vi "UHR-Fleezers Control (host) - 11.9c.vi"() -> ()   [LabVIEW 2014] (continued)
                              n670 = flat-sequence {
                                tunnel: w977 -> [w980]
                                tunnel: [w979] -> w976
                                tunnel: ["N Array El"] -> w975
                                tunnel: w976 -> [w994]
                                tunnel: w975 -> [w990]
                                frame #0 {
                                n671 = Multiply(x="Yank Delay (s)", y=1000.0) -> (x*y=w983:dbl)
                                n672 = Quotient & Remainder(x=w980, y="N Array El") -> (x-y*floor(x/y)=w979:u8)  [unwired: 1 out]
                                n673 = Wait (ms)(milliseconds to wait=w983) -> ()  [unwired: 1 out]
                                }
                                frame #1 {
                                n674 = Random Number (0-1)() -> (number: 0 to 1=w991:dbl)
                                n675 = Multiply(x=w990, y=w991) -> (x*y=w989:dbl)
                                n676 = Round Toward -Infinity(1:w989) -> (0:w988:dbl)
                                n677 = Select(t=w988, s="Random Choice", f=w994) -> (s? t:f=w992:dbl)
                                n678 = Select(t="Yank to Trap D (MHz)", s="Yank to which?", f="Yank to SP") -> (s? t:f=w985:dbl[])
                                n679 = Index Array(array=w985, index=w992) -> (element=w995:dbl)
                                n680 = case shown="False" "Yank to which?" {
                                tunnel: w995 -> [w996 w1023]
                                frame False {
                                n681 = flat-sequence {
                                tunnel: w996 -> [w997]
                                frame #0 {
                                n682 = property on="Trap Pos FB SP" class="DigNum (strict)"("Val(Sgnl)"=w997) -> ()  [unwired: 2 in, 2 out]
                                }
                                frame #1 {
                                n683 = Wait (ms)(milliseconds to wait=u32 700) -> ()  [unwired: 1 out]
                                }
                                frame #2 {
                                n684 = local read "Action (%)"() -> (w1002:dbl)
                                n685 = Absolute Value(x=w1002) -> (abs(x)=w1001:dbl)
                                n686 = Greater?(x=w1001, y=70.0) -> (0:w999:bool)
                                n687 = property on="Remove Action Offset" class="Bool (strict)"("Val(Sgnl)"=w999) -> ()  [unwired: 2 in, 2 out]
                                }
                                frame #3 {
                                n688 = for {
                                N: 4 -> [_]
                                n689 = flat-sequence {
                                frame #0 {
                                n690 = Wait (ms)(milliseconds to wait=u32 500) -> ()  [unwired: 1 out]
                                }
                                frame #1 {
                                n691 = local read "Action (%)"() -> (w1008:dbl)
                                n692 = Absolute Value(x=w1008) -> (abs(x)=w1007:dbl)
                                n693 = Greater?(x=w1007, y=70.0) -> (0:w1005:bool)
                                n694 = property on="Remove Action Offset" class="Bool (strict)"("Val(Sgnl)"=w1005) -> ()  [unwired: 2 in, 2 out]
                                }
                                }
                                }
                                }
                                frame #4 {
                                n695 = local read "Shift confocal"() -> (w1012:bool)
                                n696 = local read "Mean"() -> (w1015:dbl)
                                n697 = Greater?(x=w1015, y=11.0) -> (0:w1011:bool)
                                n698 = Not(x=w1011) -> (.not. x?=w1010:bool)
                                n699 = And(x=w1010, y=w1012) -> (x .and. y?=w1009:bool)
                                n700 = And(x=w1011, y=w1012) -> (x .and. y?=w1013:bool)
                                n701 = case shown="True" w1013 {
                                frame False {
                                }
                                frame True {
                                n702 = local read "Confocal X 2 (V)"() -> (w1018:dbl)
                                n703 = local read "Confocal Y 2 (V)"() -> (w1019:dbl)
                                n704 = property on="AO2" class="Slide (strict)"("Val(Sgnl)"=w1018) -> ()  [unwired: 2 in, 2 out]
                                n705 = property on="AO1" class="Slide (strict)"("Val(Sgnl)"=w1019) -> ()  [unwired: 2 in, 2 out]
                                }
                                }
                                n706 = case shown="True" w1009 {
                                frame False {
                                }
                                frame True {
                                n707 = local read "Confocal X 1 (V)"() -> (w1016:dbl)
                                n708 = local read "Confocal Y 1 (V)"() -> (w1017:dbl)
                                n709 = property on="AO1" class="Slide (strict)"("Val(Sgnl)"=w1017) -> ()  [unwired: 2 in, 2 out]
                                n710 = property on="AO2" class="Slide (strict)"("Val(Sgnl)"=w1016) -> ()  [unwired: 2 in, 2 out]
                                }
                                }
                                }
                                frame #5 {
                                n711 = Wait (ms)(milliseconds to wait=u32 1500) -> ()  [unwired: 1 out]
                                }
                                frame #6 {
                                n712 = property on="Remove Offset" class="Bool (strict)"("Val(Sgnl)"=TRUE ("Value (Signaling)")) -> ()  [unwired: 2 in, 2 out]
                                n713 = property on="Rem fb disp offset" class="Bool (strict)"("Val(Sgnl)"=TRUE ("Value (Signaling)")) -> ()  [unwired: 2 in, 2 out]
                                }
                                }
                                }
                                frame True {
                                n714 = flat-sequence {
                                tunnel: w1023 -> [w1024]
                                frame #0 {
                                n715 = property on="Trap D (MHz)" class="DigNum (strict)"("Val(Sgnl)"=w1024) -> ()  [unwired: 2 in, 2 out]
                                }
                                frame #1 {
                                n716 = Wait (ms)(milliseconds to wait=u32 500) -> ()  [unwired: 1 out]
                                }
                                frame #2 {
                                n717 = local read "Shift confocal"() -> (w1028:bool)
                                n718 = local read "Mean"() -> (w1026:dbl)
                                n719 = Greater?(x=w1026, y=11.0) -> (0:w1029:bool)
                                n720 = Not(x=w1029) -> (.not. x?=w1030:bool)
                                n721 = And(x=w1030, y=w1028) -> (x .and. y?=w1032:bool)
                                n722 = And(x=w1029, y=w1028) -> (x .and. y?=w1031:bool)
                                n723 = case shown="True" w1031 {
                                frame False {
                                }
                                frame True {
                                n724 = local read "Confocal Y 2 (V)"() -> (w1036:dbl)
                                n725 = local read "Confocal X 2 (V)"() -> (w1035:dbl)
                                n726 = property on="AO1" class="Slide (strict)"("Val(Sgnl)"=w1036) -> ()  [unwired: 2 in, 2 out]
                                n727 = property on="AO2" class="Slide (strict)"("Val(Sgnl)"=w1035) -> ()  [unwired: 2 in, 2 out]
                                }
                                }
                                n728 = case shown="True" w1032 {
                                frame False {
                                }
                                frame True {
                                n729 = local read "Confocal X 1 (V)"() -> (w1033:dbl)
                                n730 = local read "Confocal Y 1 (V)"() -> (w1034:dbl)
                                n731 = property on="AO2" class="Slide (strict)"("Val(Sgnl)"=w1033) -> ()  [unwired: 2 in, 2 out]
                                n732 = property on="AO1" class="Slide (strict)"("Val(Sgnl)"=w1034) -> ()  [unwired: 2 in, 2 out]
                                }
                                }
                                }
                                }
                                }
                                }
                                }
                              }
                            }
                            frame "Raster" {
                              n733 = property on="Trap Raster Scan" class="Bool (strict)"("Val(Sgnl)"=TRUE ("Value (Signaling)")) -> ()  [unwired: 2 in, 2 out]
                            }
                          }
                          n734 = local read "Time (s)"() -> (w969:dbl)
                          "Fl. High" <- TRUE ("Yanking")
                        }
                        frame #1 {
                          n735 = local read "Auto F Reset"() -> (w1038:bool)
                          n736 = case shown="True" w1038 {
                            tunnel: w1043 -> [_ w1047]
                            tunnel: w1042 -> [_ w1046]
                            tunnel: w1041 -> [_ w1045]
                            tunnel: w1039 -> [_ w1044]
                            frame False {
                            }
                            frame True {
                              n737 = node-c288() -> (w1049:T22)  [unwired: 4 out]
                              n738 = timed-loop {
                                timing: w1049 -> [_]
                                timing-out: [_] -> w1048
                                tunnel: w1047 -> [w1067]
                                tunnel: w1046 -> [w1066]
                                tunnel: w1045 -> [w1065]
                                tunnel: w1044 -> [w1064]
                                stop <- w1050 stop-if-true
                                n739 = node-c288() -> ()  [unwired: 2 out]
                                n740 = local read "Fl. D Thresh. (kHz)"() -> (w1058:dbl)
                                n741 = local read "Fl. Triggered..."() -> (w1063:bool)
                                n742 = local read "Delta Fl. 1"() -> (w1054:dbl)
                                n743 = local read "Delta Fl. 2"() -> (w1052:dbl)
                                n744 = local read "Stop All"() -> (w1061:bool)
                                n745 = local read "APD to Watch"() -> (w1053:bool)
                                n746 = Select(t=w1054, s=w1053, f=w1052) -> (s? t:f=w1051:dbl)
                                n747 = Not(x=w1063) -> (.not. x?=w1062:bool)
                                n748 = Multiply(x=w1058, y=1000.0) -> (x*y=w1057:dbl)
                                n749 = Negate(x=w1057) -> (-x=w1056:dbl)
                                n750 = Less?(x=w1051, y=w1056) -> (x < y?=w1060:bool)
                                n751 = Compound Arithmetic op=OR(w1060, w1061, w1062, "Reset Force") -> (w1050:bool)
                                n752 = case shown="True" w1050 {
                                tunnel: w1067 -> [_ w1082]
                                tunnel: w1066 -> [_ w1081]
                                tunnel: w1065 -> [_ w1071]
                                tunnel: w1064 -> [_ w1073]
                                frame False {
                                }
                                frame True {
                                n753 = local read "Time (s)"() -> (w1072:dbl)
                                n754 = case shown="\"Yank\"" w1081 {
                                tunnel: w1082 -> [_ w1085]
                                tunnel: w1073 -> [_ w1083]
                                frame "Image", Default {
                                }
                                frame "Yank" {
                                n755 = flat-sequence {
                                tunnel: [w1091] -> w1086
                                tunnel: w1085 -> [w1091]
                                tunnel: [w1087] -> w1084
                                tunnel: w1083 -> [w1087]
                                tunnel: w1086 -> [w1094]
                                tunnel: w1084 -> [w1092]
                                frame #0 {
                                n756 = local read "Yank Delay (s)"() -> (w1090:dbl)
                                n757 = Multiply(x=w1090, y=1000.0) -> (x*y=w1088:dbl)
                                n758 = Wait (ms)(milliseconds to wait=w1088) -> ()  [unwired: 1 out]
                                }
                                frame #1 {
                                n759 = local read "Yank to which?"() -> (w1093:bool)
                                n760 = case shown="False" w1093 {
                                tunnel: w1094 -> [_ w1122]
                                tunnel: w1092 -> [w1095 _]
                                frame False {
                                n761 = flat-sequence {
                                tunnel: w1095 -> [w1096]
                                frame #0 {
                                n762 = property on="Trap Pos FB SP" class="DigNum (strict)"("Val(Sgnl)"=w1096) -> ()  [unwired: 2 in, 2 out]
                                }
                                frame #1 {
                                n763 = Wait (ms)(milliseconds to wait=u32 700) -> ()  [unwired: 1 out]
                                }
                                frame #2 {
                                n764 = local read "Action (%)"() -> (w1101:dbl)
                                n765 = Absolute Value(x=w1101) -> (abs(x)=w1100:dbl)
                                n766 = Greater?(x=w1100, y=70.0) -> (0:w1098:bool)
                                n767 = property on="Remove Action Offset" class="Bool (strict)"("Val(Sgnl)"=w1098) -> ()  [unwired: 2 in, 2 out]
                                }
                                frame #3 {
                                n768 = for {
                                N: 4 -> [_]
                                n769 = flat-sequence {
                                frame #0 {
                                n770 = Wait (ms)(milliseconds to wait=u32 500) -> ()  [unwired: 1 out]
                                }
                                frame #1 {
                                n771 = local read "Action (%)"() -> (w1107:dbl)
                                n772 = Absolute Value(x=w1107) -> (abs(x)=w1106:dbl)
                                n773 = Greater?(x=w1106, y=70.0) -> (0:w1104:bool)
                                n774 = property on="Remove Action Offset" class="Bool (strict)"("Val(Sgnl)"=w1104) -> ()  [unwired: 2 in, 2 out]
                                }
                                }
                                }
                                }
                                frame #4 {
                                n775 = local read "Shift confocal"() -> (w1112:bool)
                                n776 = local read "Mean"() -> (w1114:dbl)
                                n777 = Greater?(x=w1114, y=11.0) -> (0:w1111:bool)
                                n778 = Not(x=w1111) -> (.not. x?=w1110:bool)
                                n779 = And(x=w1111, y=w1112) -> (x .and. y?=w1109:bool)
                                n780 = And(x=w1110, y=w1112) -> (x .and. y?=w1108:bool)
                                n781 = case shown="True" w1109 {
                                frame False {
                                }
                                frame True {
                                n782 = local read "Confocal Y 2 (V)"() -> (w1118:dbl)
                                n783 = local read "Confocal X 2 (V)"() -> (w1117:dbl)
                                n784 = property on="AO2" class="Slide (strict)"("Val(Sgnl)"=w1117) -> ()  [unwired: 2 in, 2 out]
                                n785 = property on="AO1" class="Slide (strict)"("Val(Sgnl)"=w1118) -> ()  [unwired: 2 in, 2 out]
                                }
                                }
                                n786 = case shown="True" w1108 {
                                frame False {
                                }
                                frame True {
                                n787 = local read "Confocal X 1 (V)"() -> (w1115:dbl)
                                n788 = local read "Confocal Y 1 (V)"() -> (w1116:dbl)
                                n789 = property on="AO1" class="Slide (strict)"("Val(Sgnl)"=w1116) -> ()  [unwired: 2 in, 2 out]
                                n790 = property on="AO2" class="Slide (strict)"("Val(Sgnl)"=w1115) -> ()  [unwired: 2 in, 2 out]
                                }
                                }
                                }
                                frame #5 {
                                n791 = Wait (ms)(milliseconds to wait=u32 1500) -> ()  [unwired: 1 out]
                                }
                                frame #6 {
                                n792 = property on="Rem fb disp offset" class="Bool (strict)"("Val(Sgnl)"=TRUE ("Value (Signaling)")) -> ()  [unwired: 2 in, 2 out]
                                n793 = property on="Remove Offset" class="Bool (strict)"("Val(Sgnl)"=TRUE ("Value (Signaling)")) -> ()  [unwired: 2 in, 2 out]
                                }
                                }
                                }
                                frame True {
                                n794 = flat-sequence {
                                tunnel: w1122 -> [w1123]
                                frame #0 {
                                n795 = property on="Trap D (MHz)" class="DigNum (strict)"("Val(Sgnl)"=w1123) -> ()  [unwired: 2 in, 2 out]
                                }
                                frame #1 {
                                n796 = Wait (ms)(milliseconds to wait=u32 500) -> ()  [unwired: 1 out]
                                }
                                frame #2 {
                                n797 = local read "Shift confocal"() -> (w1129:bool)
                                n798 = local read "Mean"() -> (w1131:dbl)
                                n799 = Greater?(x=w1131, y=11.0) -> (0:w1128:bool)
                                n800 = Not(x=w1128) -> (.not. x?=w1127:bool)
                                n801 = And(x=w1128, y=w1129) -> (x .and. y?=w1126:bool)
                                n802 = And(x=w1127, y=w1129) -> (x .and. y?=w1125:bool)
                                n803 = case shown="True" w1126 {
                                frame False {
                                }
                                frame True {
                                n804 = local read "Confocal Y 2 (V)"() -> (w1135:dbl)
                                n805 = local read "Confocal X 2 (V)"() -> (w1134:dbl)
                                n806 = property on="AO2" class="Slide (strict)"("Val(Sgnl)"=w1134) -> ()  [unwired: 2 in, 2 out]
                                n807 = property on="AO1" class="Slide (strict)"("Val(Sgnl)"=w1135) -> ()  [unwired: 2 in, 2 out]
                                }
                                }
                                n808 = case shown="True" w1125 {
                                frame False {
                                }
                                frame True {
                                n809 = local read "Confocal Y 1 (V)"() -> (w1133:dbl)
                                n810 = local read "Confocal X 1 (V)"() -> (w1132:dbl)
                                n811 = property on="AO2" class="Slide (strict)"("Val(Sgnl)"=w1132) -> ()  [unwired: 2 in, 2 out]
                                n812 = property on="AO1" class="Slide (strict)"("Val(Sgnl)"=w1133) -> ()  [unwired: 2 in, 2 out]
                                }
                                }
                                }
                                }
                                }
                                }
                                }
                                }
                                }
                                }
                                n813 = local read "Messages"() -> (w1080:string)
                                n814 = Subtract(x=w1072, y=w1071) -> (x-y=w1078:dbl)
                                "Duration (s)" <- w1078
                                n815 = Number To Decimal String(number=w1078, width (-)=i16 0) -> (decimal integer string=w1076:string)
                                n816 = Concatenate Strings(w1076, " s fluorescence event." ("string")) -> (w1074:string)
                                n817 = call "Update messages.vi"("Message to add"=w1074, "Old message string"=w1080) -> ("New message string"=w1079:string)
                                n818 = local write "Reset Force"(FALSE ("Reset Force")) -> ()
                                n819 = local write "Waiting"(TRUE ("Waiting")) -> ()
                                n820 = local write "Messages"(w1079) -> ()
                                n821 = local write "Fl. High"(FALSE ("Fl. High")) -> ()
                                n822 = call <vilib>:"Beep.vi"() -> ()  [unwired: 3 in, 9 out]
                                }
                                }
                                n823 = node-c288() -> ()  [unwired: 2 out]
                              }
                              n824 = node-c288(w1048) -> ()  [unwired: 1 out]
                            }
                          }
                        }
                      }
                      n825 = local read "Trap Pos FB SP"() -> (w956:fxp<+/-,16,1>)
                      n826 = local read "Trap D (MHz)"() -> (w961:dbl)
                    }
                  }
                }
                frame #1 {
                  n827 = local read "Stop All"() -> (w1145:bool)
                  n828 = local read "Fl. Triggered..."() -> (w1143:bool)
                  n829 = Not(x=w1143) -> (.not. x?=w1144:bool)
                  n830 = Or(x=w1144, y=w1145) -> (x .or. y?=w1142:bool)
                }
              }
              n831 = case shown="True" w731 {
                frame False {
                }
                frame True {
                  n832 = local read "Confocal Y 1 (V)"() -> (w741:dbl)
                  n833 = local read "Confocal X 1 (V)"() -> (w740:dbl)
                  n834 = property on="AO2" class="Slide (strict)"("Val(Sgnl)"=w740) -> ()  [unwired: 2 in, 2 out]
                  n835 = property on="AO1" class="Slide (strict)"("Val(Sgnl)"=w741) -> ()  [unwired: 2 in, 2 out]
                }
              }
              n836 = case shown="True" w731 {
                frame False {
                }
                frame True {
                  w739 = FALSE ("Fl. High")
                  n837 = local write "Waiting"(w739) -> ()
                  n838 = local write "Fl. High"(w739) -> ()
                }
              }
              n839 = node-c288() -> ()  [unwired: 2 out]
            }
            n840 = node-c288(w729) -> ()  [unwired: 1 out]
          }
        }
      }
      event "Stop All": Value Change {
        n841 = event-data() -> ()  [unwired: 7 out]
        n842 = local read "Stop All"() -> (w1150:bool)
      }
    }
    n843 = node-c288() -> ()  [unwired: 2 out]
  }
  n844 = property on="Saved trap pos" class="WFGraph (strict)"("Visible"=TRUE) -> ()  [unwired: 2 in, 2 out]
  n845 = property on="Trap Delta Graph" class="WFGraph (strict)"("Visible"=FALSE) -> ()  [unwired: 2 in, 2 out]
  n846 = local write "Trap pos"(TRUE ("Trap pos")) -> ()
  n847 = node-c288(2 ("Processor")) -> (w120:T22)  [unwired: 3 out]
  n848 = timed-loop "Control parameters (event loop)" {
    tunnel: w32 -> [w1159]
    shift-right: [w1158] -> _
    shift-left: errorcluster {"status"=FALSE, "code"=0, "source"=""} ("error out") -> [w1157]
    tunnel: [w1156] -> _
    timing: w120 -> [_]
    timing-out: [_] -> w119
    tunnel: w93 -> [w1155]
    tunnel: w36 -> [w1154]
    tunnel: w35 -> [w1153]
    tunnel: w34 -> [w1152]
    tunnel: w33 -> [w1151]
    stop <- w1156 stop-if-true
    n849 = node-c288() -> ()  [unwired: 2 out]
    n850 = event shown="[30] \"Invert APD Gate\", \"APD Gate ON Count\", \"APD Gate OFF Count\", \"APD Gate\", \"APD Integration Time (s)\", \"APD 1 AO Mult.\", \"APD 2 AO Mult.\", \"Duty frequency (ON 1/N cycles)\": Value Change" {
      selector: _ -> [_ _ _ _ _ _ _ _ _ _ _ _ _ _ _ _ _ _ _ _ _ _ _ _ _ _ _ _ _ _ _ _ _ _ _ _ _ _ _ _ _ _ _ _ _ _ _ _ _ _ _ _ _ _ _ _ _ _ _ _ _ _ _ _ _ _ _ _ _ _ _ _ _ _ _ _ _ _ _ _]
      dyn-events: _ -> [_ _ _ _ _ _ _ _ _ _ _ _ _ _ _ _ _ _ _ _ _ _ _ _ _ _ _ _ _ _ _ _ _ _ _ _ _ _ _ _ _ _ _ _ _ _ _ _ _ _ _ _ _ _ _ _ _ _ _ _ _ _ _ _ _ _ _ _ _ _ _ _ _ _ _ _ _ _ _ _]
      timeout: _ -> [_ _ _ _ _ _ _ _ _ _ _ _ _ _ _ _ _ _ _ _ _ _ _ _ _ _ _ _ _ _ _ _ _ _ _ _ _ _ _ _ _ _ _ _ _ _ _ _ _ _ _ _ _ _ _ _ _ _ _ _ _ _ _ _ _ _ _ _ _ _ _ _ _ _ _ _ _ _ _ _]
      tunnel: w1159 -> [w1197 _ _ _ w1235 _ w1257 _ _ _ _ w1323 _ _ w1366 w1372 w1377 w1383 w1419 w1441 w1450 _ w1467 w1471 w1482 w1493 w1504 w1521 w1532 w1543 w1570 w1664 w1671 w1709 _ _ w1769 w1773 w1784 w1788 w1792 _ w1800 _ _ _ _ _ _ _ _ _ _ _ _ _ _ _ _ _ w2181 _ w2198 _ w2205 w2223 _ w2230 w2238 w2253 w2264 w2270 _ w2279 _ w2298 _ _ _ w2373]
      tunnel: [w1196 _ _ _ w1225 _ w1256 _ _ w1288 _ w1302 _ _ w1365 w1368 w1374 w1380 w1418 w1439 w1449 _ w1465 _ w1476 w1487 w1498 w1515 w1526 w1537 w1568 w1662 w1669 w1707 _ _ w1767 w1771 w1774 w1786 w1790 _ w1798 _ _ _ _ _ _ _ _ _ _ _ _ _ _ _ _ _ w2179 _ _ _ _ w2220 _ _ _ _ _ _ _ _ _ _ _ _ _ w2371] -> w1158
      tunnel: w1157 -> [w1195 _ _ _ w1234 _ w1255 _ _ w1288 _ w1322 _ _ w1364 w1367 w1373 w1379 w1417 w1440 w1448 _ w1466 w1470 w1481 w1492 w1503 w1520 w1531 w1542 w1569 w1663 w1670 w1708 _ _ w1768 w1772 w1783 w1787 w1791 _ w1799 _ _ _ _ _ _ _ _ _ _ _ _ _ _ _ _ _ w2180 _ w2197 _ w2204 w2222 _ w2229 w2237 w2252 w2263 w2269 _ w2278 _ w2297 _ _ _ w2372]
      tunnel: [_ _ _ _ _ _ _ _ _ w1287 _ _ _ _ _ _ _ _ _ _ _ _ _ _ _ _ _ _ _ _ _ _ _ _ _ _ _ _ _ _ _ _ _ _ _ _ _ _ _ _ _ _ _ _ _ _ _ _ _ _ _ _ _ _ _ _ _ _ _ _ _ _ _ _ _ _ _ _ _ _] -> w1156
      tunnel: [_ _ _ _ _ _ _ "Round T1 X" _ _ _ _ _ _ _ _ _ _ _ _ _ _ _ _ _ _ _ _ _ _ _ _ _ _ _ _ _ _ _ _ _ _ _ _ _ _ _ _ _ _ _ _ _ _ _ _ _ _ _ _ _ _ _ _ _ _ _ _ _ _ _ _ _ _ _ _ _ _ _ _] -> _
      tunnel: [_ _ _ "Adjust Scale\nto Mean" _ _ _ _ _ _ _ _ _ _ _ _ _ _ _ _ _ _ "Test ttrig" _ _ _ _ _ _ _ _ _ _ _ _ _ _ _ _ _ _ _ _ _ _ _ _ _ _ _ "Flush Sample" "Flush Pump 3" "Flush Pump 1" "Clear Volume" _ _ _ _ _ _ _ _ _ _ _ _ _ _ _ _ _ _ _ _ _ _ _ _ _ _] -> _
      tunnel: [_ _ _ _ _ _ _ _ "Round T2 X" _ "Delayed Interlace Start" _ _ _ _ _ _ _ _ _ _ _ _ _ _ _ _ _ _ _ _ _ _ _ _ _ _ _ _ _ _ _ _ _ _ _ _ _ _ _ _ _ _ _ _ _ _ _ _ _ _ _ _ _ _ _ _ _ _ _ _ _ _ _ _ _ _ _ _ _] -> _
      tunnel: w1155 -> [_ _ _ _ _ _ _ _ _ _ _ _ _ _ _ _ _ _ _ _ _ _ _ _ _ _ _ _ _ _ _ _ _ _ _ _ _ _ _ _ _ _ _ _ _ _ w1958 w1976 w1983 w1988 w1994 _ _ w2093 _ _ _ _ _ _ _ _ _ _ _ _ _ _ _ _ _ _ _ _ _ _ _ _ _ _]
      tunnel: w1154 -> [_ _ _ _ _ _ _ _ _ _ _ _ _ _ _ _ _ _ _ _ _ _ _ _ _ _ _ _ _ _ _ _ _ _ _ _ _ _ _ _ _ _ _ _ w1874 _ _ _ _ _ _ w2024 _ _ w2100 _ w2109 _ w2123 _ _ _ _ _ _ _ _ _ _ _ _ _ _ _ _ _ _ _ _ _]
      tunnel: w1153 -> [_ _ _ _ _ _ _ _ _ _ _ _ _ _ _ _ _ _ _ _ _ _ _ _ _ _ _ _ _ _ _ _ _ _ _ _ _ _ _ _ _ _ _ _ _ _ _ _ _ _ _ _ _ _ _ _ _ _ _ _ _ _ _ _ _ _ _ _ _ _ _ _ _ _ _ _ _ _ _ _]
      tunnel: w1152 -> [_ _ _ _ _ _ _ _ _ _ _ _ _ _ _ _ _ _ _ _ _ _ _ _ _ _ _ _ _ _ _ _ _ _ _ _ _ _ _ _ _ _ _ w1811 _ _ _ _ _ _ _ _ w2054 _ _ w2105 _ w2116 _ w2148 _ _ _ _ _ _ _ _ _ _ _ _ _ _ _ _ _ _ _ _]
      tunnel: w1151 -> [_ _ _ _ _ _ _ _ _ _ _ _ _ _ _ _ _ _ _ _ _ _ _ _ _ _ _ _ _ _ _ _ _ _ _ _ _ _ _ _ _ _ _ _ _ _ _ _ _ _ _ _ _ _ _ _ _ _ _ _ _ _ _ _ _ _ _ _ _ _ _ _ _ _ _ _ _ _ _ _]
      event "AI Count (ticks)", "Sets to FIFO (Traps)", "Save ave N", "FPGA Ave.", "# Samples/channel", "N sets to save": Value Change {
        # "So that if 'Save ave N' is updated, the AOD scanning code updates too."
        n851 = event-data() -> ()  [unwired: 6 out]
        n852 = local read "AI Count (ticks)"() -> (w1177:u32)
        n853 = Boolean To (0,1)(Boolean="Sets to FIFO (Traps)") -> (0, 1=w1187:cluster{"Set 1":i16, "Set 2":i16, "Set 3":i16})
        n854 = Cluster To Array(cluster=w1187) -> (array=w1186:i16[])
        n855 = xnode "Read/Write Control"("FPGA VI Reference In"=w1197, "error in"=w1195, "ai count"=w1177, "AI1 Sets to FIFO"="Sets to FIFO (Traps)", "N of AI1 Int Acq Sets"="N Acq Sets (Traps + Fl.)") -> ("error out"=w1196:errorcluster)  [unwired: 1 out]
        n856 = To Unsigned Long Integer(number=w1186) -> (unsigned 32bit integer=w1166:u32[])
        n857 = local read "Scan steps (AOD)"() -> (w1188:u64)
        n858 = Multiply(x=w1177, y="N Acq Sets (Traps + Fl.)") -> (x*y=w1175:u32)
        n859 = Divide(x=40000000.0, y=w1177) -> (x/y=w1169:dbl)
        "AI rate (Hz)" <- w1169
        "Ave. Rate (Hz)" <- w1169
        n860 = Add Array Elements(numeric array=w1166) -> (sum=w1178:u32)
        "Trap Sets" <- w1178
        n861 = Reciprocal(x=w1169) -> (1/x=→"Ave. Period (s)":dbl)
        n862 = property on="Scan steps (AOD)" class="DigNum (strict)"("Val(Sgnl)"=w1188) -> ()  [unwired: 2 in, 2 out]
        n863 = Divide(x=w1169, y="N Acq Sets (Traps + Fl.)") -> (x/y=w1192:dbl)
        "Data Rate (Hz)" <- w1192
        n864 = Reciprocal(x=w1192) -> (1/x=→"Data Period (s)":dbl)
        n865 = local read "Save ave N"() -> (w1191:dbl)
        n866 = Divide(x=w1192, y=w1191) -> (x/y=w1190:dbl)
        "Save Data Rate (Hz)" <- w1190
        n867 = Reciprocal(x=w1190) -> (1/x=→"Save Data Period (s)":dbl)
        n868 = Multiply(x=w1175, y="# Samples/trap") -> (x*y=w1173:u32)
        "Counts/DMA" <- w1173
        n869 = property on="Trap Disp. Downsample" class="DigNum (strict)"("Maximum"="# Samples/trap") -> ()  [unwired: 2 in, 2 out]
        n870 = Multiply(x=w1178, y="# Samples/trap") -> (x*y=w1167:u32)
        "# Samples/channel" <- w1167
        n871 = Multiply(x=w1167, y=u32 8) -> (x*y=→"Trap AI Elements/DMA read":u32)
        n872 = local read "APD Int. Count"() -> (w1174:u32)
        n873 = Multiply(x=w1167, y=u32 3) -> (x*y=→"Trap Pos Elements/DMA read":u32)
        n874 = Divide(x=w1173, y=w1174) -> (x/y=w1164:dbl)
        "APD Samples/FIFO Acq." <- w1164
        n875 = Divide(x=w1173, y=40000000.0) -> (x/y=w1171:dbl)
        "DMA Update Period (s)" <- w1171
        n876 = Multiply(x=2.0, y=w1164) -> (x*y=→"APD Elements/DMA read":dbl)
        n877 = property on="APD Disp. Downsample" class="DigNum (strict)"("Maximum"=w1164) -> ()  [unwired: 2 in, 2 out]
        n878 = local read "N sets to save"() -> (w1184:u32)
        n879 = Multiply(x=w1171, y=w1184) -> (x*y=→"Total Time (s)":dbl)
        "FPGA Averaging" <- FALSE ("FPGA Averaging")
      }
      event "Remove Offset": Value Change {
        n880 = event-data() -> ()  [unwired: 7 out]
        n881 = local write "Remove Offset"(FALSE ("Remove Offset")) -> ()
        n882 = local read "Bead Mean (nm)"() -> (w1199:dbl)
        n883 = local read "Offset (nm)"() -> (w1200:dbl)
        n884 = Add(x=w1199, y=w1200) -> (x+y=w1198:dbl)
        n885 = local write "Offset (nm)"(w1198) -> ()
        n886 = disable-structure shown="Disabled" {
          frame Disabled {
            n887 = local read "Bead Mean (nm)"() -> (w1205:dbl)
            n888 = Add(y=w1205) -> (x=w1204:dbl, x+y=w1203:dbl)
            n889 = Subtract(x=w1205, y=w1204) -> (x-y=w1202:dbl)
            n890 = property on="Bead Separation" class="WFChart (strict)"("YScale.Minimum"=w1202) -> ()  [unwired: 2 in, 2 out]
            n891 = property on="Bead Separation" class="WFChart (strict)"("YScale.Maximum"=w1203) -> ()  [unwired: 2 in, 2 out]
          }
          frame Enabled {
          }
        }
      }
      event "Detector Type": Value Change {
        n892 = event-data() -> ()  [unwired: 7 out]
        n893 = local read "AI labels"() -> (w1206:string[])
        n894 = property on="High Res. Display" class="Ring (strict)"("Strings []"=w1206) -> ()  [unwired: 2 in, 2 out]
        n895 = Build Array (concatenate)(w1206, "none") -> (w1207:string[])
        n896 = property on="FFT 1 Choice 1" class="Ring (strict)"("Strings []"=w1207) -> ()  [unwired: 2 in, 2 out]
        n897 = property on="FFT 1 Choice 2" class="Ring (strict)"("Strings []"=w1207) -> ()  [unwired: 2 in, 2 out]
        n898 = property on="FFT 2 Choice 1" class="Ring (strict)"("Strings []"=w1207) -> ()  [unwired: 2 in, 2 out]
        n899 = property on="FFT 2 Choice 2" class="Ring (strict)"("Strings []"=w1207) -> ()  [unwired: 2 in, 2 out]
        n900 = Bundle("APD 1", "APD 2") -> (w1210:cluster{string, string})  [unwired: 1 out]
        n901 = Cluster To Array(cluster=w1210) -> (array=w1208:string[])
        n902 = Build Array (concatenate)(w1208, w1207) -> (w1212:string[])
        n903 = Array Size(array=w1212) -> (size(s)=w1213:i32)
        n904 = property on="Signals to Plot" class="LstBox (strict)"("Item Names"=w1212) -> ()  [unwired: 2 in, 2 out]
        n905 = property on="Signals to Plot" class="LstBox (strict)"("Number of Rows"=w1213) -> ()  [unwired: 2 in, 2 out]
        n906 = property on="All Signals" class="WFChart (strict)"("LegNumRows"=w1213) -> ()  [unwired: 2 in, 2 out]
      }
      event "Adjust Scale\nto Mean": Value Change {
        n907 = event-data() -> ()  [unwired: 7 out]
        n908 = local read "APD 1 Rate (Hz)"() -> (w1222:dbl)
        n909 = Multiply(x=1000.0, y="Above (kHz)") -> (x*y=w1220:dbl)
        n910 = Multiply(x=1000.0, y="Below (kHz)") -> (x*y=w1218:dbl)
        n911 = Add(x=w1220, y=w1222) -> (x+y=w1215:dbl)
        n912 = Subtract(x=w1222, y=w1218) -> (x-y=w1216:dbl)
        n913 = property on="APD Chart" class="WFChart (strict)"("YScale.Minimum"=w1216) -> ()  [unwired: 2 in, 2 out]
        n914 = property on="APD Chart" class="WFChart (strict)"("YScale.Maximum"=w1215) -> ()  [unwired: 2 in, 2 out]
      }
      event "Phase adj. (AI1)", "+ phase (AI1)", "- phase (AI1)": Value Change {
        n915 = event-data() -> ()  [unwired: 7 out]
        n916 = Negate(x="Phase adj. (AI1)") -> (-x=w1232:i16)
        n917 = Select(t=w1232, s="- phase (AI1)", f="Phase adj. (AI1)") -> (s? t:f=w1231:i16)
        n918 = xnode "Read/Write Control"("FPGA VI Reference In"=w1235, "error in"=w1234, "Phase count adjustment"=w1231) -> ("FPGA VI Reference Out"=w1230:T20, "error out"=w1229:errorcluster)
        n919 = Or(x="- phase (AI1)", y="+ phase (AI1)") -> (x .or. y?=w1226:bool)
        n920 = xnode "Read/Write Control"("FPGA VI Reference In"=w1230, "error in"=w1229, "+ phase"=w1226) -> ("error out"=w1225:errorcluster)  [unwired: 1 out]
      }
      event "Signals to Plot": Double Click {
        w1238 = u32 9868950 ("Color Box")
        n921 = event-data() -> ("Row"=w1240:i32)  [unwired: 9 out]
        n922 = property on="All Signals" class="WFChart (strict)"("Active Plot"=w1240) -> (error out=w1251:errorcluster)  [unwired: 2 in, 1 out]
        n923 = property on="All Signals" class="WFChart (strict)" props=["Plot", "Visible?", "Plot", "Plot Color"](error in=w1251) -> (error out=w1250:errorcluster, "Plot.Visible?"=w1249:bool)  [unwired: 1 in, 2 out]
        n924 = Select(t=FALSE ("Plot.Visible"), s=w1249, f=TRUE ("Plot.Visible")) -> (s? t:f=w1244:bool)
        n925 = property on="All Signals" class="WFChart (strict)"(error in=w1250, "Plot.Visible?"=w1244) -> (error out=w1246:errorcluster)  [unwired: 1 in, 1 out]
        n926 = property on="All Signals" class="WFChart (strict)"(error in=w1246) -> (error out=w1241:errorcluster, "Plot.Plot Color"=w1245:u32)  [unwired: 1 in, 1 out]
        n927 = property on="Signals to Plot" class="LstBox (strict)"(error in=w1241, "Active Row"=w1240) -> (error out=w1239:errorcluster)  [unwired: 1 in, 1 out]
        n928 = Select(t=w1245, s=w1244, f=u32 0) -> (s? t:f=w1242:u32)
        n929 = property on="Signals to Plot" class="LstBox (strict)"(error in=w1239, "CellFontColor"=w1242, "SelColor"=w1238, "CellBG"=w1238, "CellFontSize"=u32 20 ("Active Row:Cell Font:Size"), "CellFontBold"=TRUE ("Active Row:Cell Font:Bold")) -> ()  [unwired: 1 in, 2 out]
      }
      event "BD 1 Frequency 1 (MHz)", "BD 1 Frequency 2 (MHz)", "BD 1 Frequency 3 (MHz)", "BD 2 Frequency 1 (MHz)", "BD 2 Frequency 2 (MHz)", "BD 2 Frequency 3 (MHz)", "Trap D (MHz)": Value Change {
        n930 = event-data() -> ("CtlRef"=w1254:refnum<vi>)  [unwired: 6 out]
        n931 = control-ref of="Trap D (MHz)"() -> (w1253:refnum<vi>)
        n932 = Equal?(x=w1253, y=w1254) -> (x = y?=w1252:bool)
        n933 = case shown="False" "Oscillate Set 1" {
          tunnel: w1257 -> [w1277 _]
          tunnel: [w1276 w1280] -> w1256
          tunnel: w1255 -> [w1275 w1280]
          tunnel: w1252 -> [w1260 _]
          frame False {
            n934 = local read "BD 1 Frequency 2 (MHz)"() -> (w1264:dbl)
            n935 = local read "BD 1 Frequency 1 (MHz)"() -> (w1262:dbl)
            n936 = Subtract(x=w1264, y="Trap D (MHz)") -> (x-y=w1261:dbl)
            n937 = Select(t=w1261, s=w1260, f=w1262) -> (s? t:f=w1259:dbl)
            n938 = local read "Y RF Frequency Limits (MHz)"() -> (w1265:T17)
            n939 = local read "X RF Frequency Limits (MHz)"() -> (w1266:T17)
            n940 = local read "BD 1 Frequency 3 (MHz)"() -> (w1278:dbl)
            n941 = local write "BD 1 Frequency 1 (MHz)"(w1259) -> ()
            n942 = local read "BD 2 Frequency 1 (MHz)"() -> (w1269:dbl)
            n943 = local read "BD 2 Frequency 2 (MHz)"() -> (w1268:dbl)
            n944 = local read "BD 2 Frequency 3 (MHz)"() -> (w1279:dbl)
            n945 = call "set RF board frequency - interlace.vi"("Board 2 Frequency Limits"=w1265, "Board 1 Frequency Limits"=w1266, "error in"=w1275, "FPGA VI Reference In"=w1277, "Board 2 Frequency 3 (MHz)"=w1279, "Board 1 Frequency 3 (MHz)"=w1278, "Board 2 Frequency 2 (MHz)"=w1268, "Board 2 Frequency 1 (MHz)"=w1269, "Board 1 Frequency 2 (MHz)"=w1264, "Board 1 Frequency 1  (MHz)"=w1259) -> ("error out"=w1276:errorcluster)  [unwired: 1 out]
            n946 = Subtract(x=w1269, y=w1268) -> (x-y=w1273:dbl)
            n947 = Subtract(x=w1259, y=w1264) -> (x-y=w1274:dbl)
            n948 = Square(x=w1273) -> (x^2=w1271:dbl)
            n949 = Square(x=w1274) -> (x^2=w1272:dbl)
            n950 = Add(x=w1272, y=w1271) -> (x+y=w1270:dbl)
            n951 = Square Root(x=w1270) -> (sqrt(x)=w1267:dbl)
            n952 = local write "Trap D (MHz)"(w1267) -> ()
            n953 = property on="Initial D (MHz)" class="DigNum (strict)"("Val(Sgnl)"=w1267) -> ()  [unwired: 2 in, 2 out]
          }
          frame True {
          }
        }
      }
      event "Round T1 X": Value Change {
        n954 = event-data() -> ()  [unwired: 7 out]
        n955 = local read "BD 1 Frequency 1 (MHz)"() -> (w1283:dbl)
        n956 = Round To Nearest(number=w1283) -> (nearest integer value=w1282:dbl)
        n957 = property on="BD 1 Frequency 1 (MHz)" class="DigNum (strict)"("Val(Sgnl)"=w1282) -> ()  [unwired: 2 in, 2 out]
      }
      event "Round T2 X": Value Change {
        n958 = event-data() -> ()  [unwired: 7 out]
        n959 = local read "BD 1 Frequency 2 (MHz)"() -> (w1285:dbl)
        n960 = Round To Nearest(number=w1285) -> (nearest integer value=w1284:dbl)
        n961 = property on="BD 1 Frequency 2 (MHz)" class="DigNum (strict)"("Val(Sgnl)"=w1284) -> ()  [unwired: 2 in, 2 out]
      }
      event "Stop All": Value Change {
        n962 = event-data() -> ()  [unwired: 7 out]
        n963 = local read "Stop All"() -> (w1287:bool)
      }
      event "Delayed Interlace Start": Value Change {
        n964 = event-data() -> ()  [unwired: 7 out]
        n965 = flat-sequence {
          frame #0 {
            n966 = Multiply(x="Delay to Interlace (s)", y=1000.0) -> (x*y=w1290:dbl)
            n967 = Wait (ms)(milliseconds to wait=w1290) -> ()  [unwired: 1 out]
          }
          frame #1 {
            n968 = property on="Laser interlacing mode (all lasers)" class="RadioBtnsControl (strict)"("Val(Sgnl)"=enum32{"Laser ON", "Laser OFF", "Interlace"}."Interlace" ("Value (Signaling)")) -> ()  [unwired: 2 in, 2 out]
          }
        }
      }
      event "BD 1 Amplitude 1 (%)", "BD 1 Amplitude 2 (%)", "BD 1 Amplitude 3 (%)", "BD 2 Amplitude 1 (%)", "BD 2 Amplitude 2 (%)", "BD 2 Amplitude 3 (%)", "Trap 1 ON", "Trap 2 ON", "Trap 3 ON", "Feedback On/Off", "All FB On/Off": Value Change {
        w1314 = i16 1 ("f")
        n969 = event-data() -> ()  [unwired: 7 out]
        n970 = local write "Trap 1 (ON/OFF)"("Trap 1 ON") -> ()
        n971 = local write "Trap 2 (ON/OFF)"("Trap 2 ON") -> ()
        n972 = Boolean To (0,1)(Boolean="Trap 3 ON") -> (0, 1=w1315:i16)
        n973 = Boolean To (0,1)(Boolean="Trap 1 ON") -> (0, 1=w1316:i16)
        n974 = Boolean To (0,1)(Boolean="Trap 2 ON") -> (0, 1=w1317:i16)
        n975 = Select(t=w1317, s="Trap ON/OFF X or Y Amp?", f=w1314) -> (s? t:f=w1312:i16)
        n976 = Select(t=w1316, s="Trap ON/OFF X or Y Amp?", f=w1314) -> (s? t:f=w1313:i16)
        n977 = Select(t=w1315, s="Trap ON/OFF X or Y Amp?", f=w1314) -> (s? t:f=w1311:i16)
        n978 = Select(t=w1314, s="Trap ON/OFF X or Y Amp?", f=w1317) -> (s? t:f=w1309:i16)
        n979 = Select(t=w1314, s="Trap ON/OFF X or Y Amp?", f=w1316) -> (s? t:f=w1310:i16)
        n980 = Select(t=w1314, s="Trap ON/OFF X or Y Amp?", f=w1315) -> (s? t:f=w1308:i16)
        n981 = And(x="All FB On/Off", y="Feedback On/Off") -> (x .and. y?=w1306:cluster{"Set 1":bool, "Set 2":bool})
        n982 = local read "BD 1 Amplitude 1 (%)"() -> (w1326:dbl)
        n983 = local read "BD 1 Amplitude 2 (%)"() -> (w1325:dbl)
        n984 = local read "BD 1 Amplitude 3 (%)"() -> (w1324:dbl)
        n985 = Unbundle By Name(w1306) -> ("Set 1"=w1301:bool, "Set 2"=w1298:bool)
        n986 = local read "Y RF Amplitude Limits (%)"() -> (w1294:T17)
        n987 = local read "X RF Amplitude Limits (%)"() -> (w1295:T17)
        n988 = local read "BD 2 Amplitude 1 (%)"() -> (w1327:dbl)
        n989 = local read "BD 2 Amplitude 2 (%)"() -> (w1328:dbl)
        n990 = local read "BD 2 Amplitude 3 (%)"() -> (w1329:dbl)
        n991 = And(x="Trap 2 ON", y=w1298) -> (x .and. y?=w1296:bool)
        n992 = And(x="Trap 1 ON", y=w1301) -> (x .and. y?=w1299:bool)
        n993 = Multiply(x=w1313, y=w1326) -> (x*y=w1321:dbl)
        n994 = Multiply(x=w1325, y=w1312) -> (x*y=w1319:dbl)
        n995 = Multiply(x=w1324, y=w1311) -> (x*y=w1320:dbl)
        n996 = Multiply(x=w1327, y=w1310) -> (x*y=w1330:dbl)
        n997 = Multiply(x=w1328, y=w1309) -> (x*y=w1331:dbl)
        n998 = Multiply(x=w1329, y=w1308) -> (x*y=w1332:dbl)
        n999 = call "set RF board amplitude - interlace.vi"("Board 2 Amplitude Limits"=w1294, "Board 1 Amplitude Limits"=w1295, "error in"=w1322, "FPGA VI Reference In"=w1323, "Board 2 Amplitude 3 (%)"=w1332, "Board 1 Amplitude 3 (%)"=w1320, "Board 2 Amplitude 2 (%)"=w1331, "Board 2 Amplitude 1 (%)"=w1330, "Board 1 Amplitude 2 (%)"=w1319, "Board 1 Amplitude 1 (%)"=w1321) -> ("error out"=w1303:errorcluster, "FPGA VI Reference Out"=w1304:T20)
        n1000 = xnode "Read/Write Control"("FPGA VI Reference In"=w1304, "error in"=w1303, "FB On/Off Set 1"=w1299, "FB On/Off Set 2"=w1296) -> ("error out"=w1302:errorcluster)  [unwired: 1 out]
      }
      event "Load parameters": Value Change {
        n1001 = event-data() -> ()  [unwired: 7 out]
        n1002 = property on="Saved AOD Raster Scan Parameter Sets" class="Arr (strict)"() -> ("Index Values"=w1343:u32[])  [unwired: 2 in, 2 out]
        n1003 = Index Array(array=w1343, index=0) -> (element=w1340:u32)
        n1004 = local write "Load parameters"(FALSE ("Load parameters")) -> ()
        n1005 = Index Array(array="Saved AOD Raster Scan Parameter Sets", index=w1340) -> (element=w1339:T27)
        n1006 = Unbundle By Name(w1339) -> ("Scan Range AOD (nm) 2"=w1338:dbl, "Step Size AOD (nm) 2"=w1337:dbl, "Scan Speed AOD (nm/s) 2"=w1336:dbl, "Number of scans (AOD) 2"=w1335:u16)
        n1007 = flat-sequence {
          tunnel: w1338 -> [w1346]
          tunnel: w1337 -> [w1345]
          tunnel: w1336 -> [w1344]
          tunnel: w1335 -> [w1347]
          frame #0 {
            n1008 = local write "Scan Speed (nm/s)"(w1344) -> ()
            n1009 = local write "Scan Range (nm)"(w1346) -> ()
            n1010 = local write "Step Size (nm)"(w1345) -> ()
          }
          frame #1 {
            n1011 = property on="Number of F/B Scans (AOD)" class="DigNum (strict)"("Val(Sgnl)"=w1347) -> ()  [unwired: 2 in, 2 out]
          }
        }
      }
      event "Trap 1 (ON/OFF)", "Trap 2 (ON/OFF)": Value Change {
        n1012 = event-data() -> ()  [unwired: 7 out]
        n1013 = property on="Trap 2 ON" class="Bool (strict)"("Val(Sgnl)"="Trap 2 (ON/OFF)") -> ()  [unwired: 2 in, 2 out]
        n1014 = property on="Trap 1 ON" class="Bool (strict)"("Val(Sgnl)"="Trap 1 (ON/OFF)") -> ()  [unwired: 2 in, 2 out]
      }
      event "DIO count 1 (ticks)", "DIO count 2 (ticks)", "DIO count 3 (ticks)", "Interlace", "Number Interlace Sets", "Not-Interlacing Set": Value Change {
        n1015 = event-data() -> ()  [unwired: 7 out]
        n1016 = local read "DIO count 3 (ticks)"() -> (w1360:u32)
        n1017 = local read "DIO count 1 (ticks)"() -> (w1362:u32)
        n1018 = local read "DIO count 2 (ticks)"() -> (w1361:u32)
        n1019 = To Unsigned Byte Integer(number="Not-Interlacing Set") -> (unsigned 8bit integer=w1351:u8)
        n1020 = Add(x=w1351, y=u8 1) -> (x+y=w1355:u8)
        n1021 = xnode "Read/Write Control"("FPGA VI Reference In"=w1366, "error in"=w1364, "DIO count 1 (ticks)"=w1362, "DIO count 2 (ticks)"=w1361, "DIO count 3 (ticks)"=w1360, "Interlace ON/OFF"="Interlace", "Number Interlace Cycles"="Number Interlace Sets", "Interlace Off Parameters"=w1355) -> ("error out"=w1365:errorcluster)  [unwired: 1 out]
        n1022 = Build Array(w1362, w1361, w1360) -> (w1353:u32[])
        n1023 = Split 1D Array(array=w1353, index="Number Interlace Sets") -> (first subarray=w1363:u32[])  [unwired: 1 out]
        n1024 = Index Array(array=w1353, index=w1351) -> (element=w1352:u32)
        n1025 = Add Array Elements(numeric array=w1363) -> (sum=w1357:u32)
        n1026 = Select(t=w1357, s="Interlace", f=w1352) -> (s? t:f=→"Total Counts (ticks)":u32)
      }
      event "Reset Feedback": Value Change {
        n1027 = event-data() -> ()  [unwired: 7 out]
        n1028 = Unbundle By Name("Reset Feedback") -> ("Set 1"=w1370:bool, "Set 2"=w1369:bool)
        n1029 = xnode "Read/Write Control"("FPGA VI Reference In"=w1372, "error in"=w1367, "FB Reset Set 1"=w1370, "FB Reset Set 2"=w1369) -> ("error out"=w1368:errorcluster)  [unwired: 1 out]
      }
      event "PID Gains": Value Change {
        n1030 = event-data() -> ()  [unwired: 7 out]
        n1031 = Unbundle By Name("PID Gains") -> ("Set 1"=w1376:T15, "Set 2"=w1375:T15)
        n1032 = xnode "Read/Write Control"("FPGA VI Reference In"=w1377, "error in"=w1373, "FB Gains Set 1"=w1376, "FB Gains Set 2"=w1375) -> ("error out"=w1374:errorcluster)  [unwired: 1 out]
      }
      event "AI2 to Setpoint", "Setpoints (V)": Value Change {
        n1033 = event-data() -> ()  [unwired: 7 out]
        n1034 = xnode "Read/Write Control"("FPGA VI Reference In"=w1383, "error in"=w1379) -> ("FPGA VI Reference Out"=w1382:T20, "error out"=w1381:errorcluster, "AI2 Y Sum Set 1"=w1390:i16, "AI2 Y Sum Set 2"=w1389:i16)
        n1035 = Cluster To Array(cluster="AI2 to Setpoint") -> (array=w1393:bool[])
        n1036 = local read "AI2 (V)"() -> (w1391:cluster{"Set 1":dbl, "Set 2":dbl})
        n1037 = Or Array Elements(Boolean array=w1393) -> (logical OR=w1394:bool)
        n1038 = Bundle By Name(cluster=w1391, "Set 1"=w1390, "Set 2"=w1389) -> (w1388:cluster{"Set 1":dbl, "Set 2":dbl})
        n1039 = Divide(x=w1388, y=3276.7) -> (x/y=w1387:cluster{"Set 1":dbl, "Set 2":dbl})
        "AI2 (V)" <- w1387
        n1040 = case shown="True" w1394 {
          tunnel: [w1397 w1414] -> w1386
          tunnel: "AI2 to Setpoint" -> [_ w1410]
          tunnel: "Setpoints (V)" -> [w1398 w1413]
          tunnel: w1387 -> [_ w1407]
          frame False {
            n1041 = Multiply(x=3276.7, y=w1398) -> (x*y=w1399:cluster{"Set 1":dbl, "Set 2":dbl})
            n1042 = To Word Integer(number=w1399) -> (16bit integer=w1397:cluster{"Set 1":i16, "Set 2":i16})
          }
          frame True {
            n1043 = Unbundle By Name(w1407) -> ("Set 1"=w1406:dbl, "Set 2"=w1405:dbl)
            n1044 = Unbundle By Name(w1413) -> ("Set 1"=w1412:dbl, "Set 2"=w1411:dbl)
            n1045 = Unbundle By Name(w1410) -> ("Set 1"=w1409:bool, "Set 2"=w1408:bool)
            n1046 = Select(t=w1406, s=w1409, f=w1412) -> (s? t:f=w1404:dbl)
            n1047 = Select(t=w1405, s=w1408, f=w1411) -> (s? t:f=w1403:dbl)
            n1048 = Bundle By Name(cluster=w1413, "Set 1"=w1404, "Set 2"=w1403) -> (w1401:cluster{"Set 1":dbl, "Set 2":dbl})
            n1049 = local write "Setpoints (V)"(w1401) -> ()
            n1050 = Multiply(x=3276.7, y=w1401) -> (x*y=w1402:cluster{"Set 1":dbl, "Set 2":dbl})
            n1051 = To Word Integer(number=w1402) -> (16bit integer=w1414:cluster{"Set 1":i16, "Set 2":i16})
          }
        }
        n1052 = Unbundle By Name(w1386) -> ("Set 1"=w1385:i16, "Set 2"=w1384:i16)
        n1053 = xnode "Read/Write Control"("FPGA VI Reference In"=w1382, "error in"=w1381, "FB Setpoint Set 1"=w1385, "FB Setpoint Set 2"=w1384) -> ("error out"=w1380:errorcluster)  [unwired: 1 out]
      }
      event "Invert laser interlacing": Value Change {
        n1054 = event-data() -> ()  [unwired: 7 out]
        n1055 = xnode "Read/Write Control"("FPGA VI Reference In"=w1419, "error in"=w1417, "Invert GI"="Invert laser interlacing", "Invert GI 2"="Invert laser interlacing", "Invert RI"="Invert laser interlacing", "Invert RI 2"="Invert laser interlacing") -> ("error out"=w1418:errorcluster)  [unwired: 1 out]
      }
      event "Green FB Setpoint (mV)", "Green FB Gains", "Green FB On/Off", "Green intensity % (FB OFF)", "Green int current ON count adj", "Red intensity % (FB OFF)": Value Change {
        n1056 = event-data() -> ()  [unwired: 7 out]
        n1057 = local read "Green FB Setpoint (mV)"() -> (w1430:dbl)
        n1058 = local read "Green intensity % (FB OFF)"() -> (w1433:dbl)
        n1059 = local read "Red intensity % (FB OFF)"() -> (w1423:dbl)
        n1060 = Multiply(x=w1430, y=3.2767) -> (x*y=w1429:dbl)
        n1061 = Multiply(x=w1433, y=655.35) -> (x*y=w1434:dbl)
        n1062 = Multiply(x=w1423, y=655.35) -> (x*y=w1421:dbl)
        n1063 = To Unsigned Word Integer(number=w1434) -> (unsigned 16bit integer=w1432:u16)
        n1064 = To Unsigned Word Integer(number=w1421) -> (unsigned 16bit integer=w1420:u16)
        n1065 = local read "Green int current ON count adj"() -> (w1437:u16)
        n1066 = local read "Green FB Gains"() -> (w1436:T15)
        n1067 = local read "Laser interlacing mode (all lasers)"() -> (w1426:enum32{"Laser ON", "Laser OFF", "Interlace"})
        n1068 = local read "Green ON/Interlacing"() -> (w1427:bool)
        n1069 = local read "Green FB On/Off"() -> (w1438:bool)
        n1070 = Equal?(x=w1426, y=enum32{"Laser ON", "Laser OFF", "Interlace"}."Interlace") -> (x = y?=w1424:bool)
        n1071 = Compound Arithmetic op=AND(w1424, w1438, w1427) -> (w1428:bool)
        n1072 = xnode "Read/Write Control"("FPGA VI Reference In"=w1441, "error in"=w1440, "Green FB Setpoint"=w1429, "Green FB On/Off"=w1428, "Current Out"=w1432, "Green int current ON count adj"=w1437, "Green FB Gains"=w1436, "RI Current Out"=w1420) -> ("error out"=w1439:errorcluster)  [unwired: 1 out]
      }
      event "Laser interlacing mode (all lasers)", "Green ON/Interlacing", "Red Laser ON/Interlacing": Value Change {
        n1073 = event-data() -> ()  [unwired: 7 out]
        n1074 = local write "Green Laser ON/OFF"("Green ON/Interlacing") -> ()
        n1075 = case shown="True" "Green ON/Interlacing" {
          tunnel: "Laser interlacing mode (all lasers)" -> [_ w1462]
          tunnel: [enum32{"Laser ON", "Laser OFF", "Interlace"}."Laser OFF" ("Green laser mode") w1462] -> w1447
          tunnel: [FALSE w1458] -> w1446
          frame False {
          }
          frame True {
            n1076 = local read "Green FB On/Off"() -> (w1459:bool)
            n1077 = Equal?(x=w1462, y=enum32{"Laser ON", "Laser OFF", "Interlace"}."Interlace") -> (x = y?=w1460:bool)
            n1078 = And(x=w1460, y=w1459) -> (x .and. y?=w1458:bool)
          }
        }
        n1079 = case shown="True" "Red Laser ON/Interlacing" {
          tunnel: "Laser interlacing mode (all lasers)" -> [_ w1453]
          tunnel: [FALSE w1454] -> _
          tunnel: [enum32{"Laser ON", "Laser OFF", "Interlace"}."Laser OFF" ("Green laser mode") w1453] -> w1442
          frame False {
          }
          frame True {
            n1080 = Equal?(x=w1453, y=enum32{"Laser ON", "Laser OFF", "Interlace"}."Interlace") -> (x = y?=w1454:bool)
          }
        }
